vi "FromBaseToMicro.vi"(11 "base":dbl) -> (3 "u":dbl format="%#_13g")   [LabVIEW 2014]
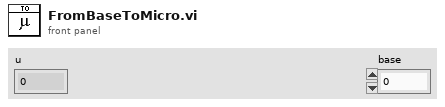
[diagram p1: front panel]
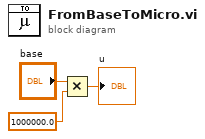
[diagram p0: block diagram]
diagram:
  n1 = Multiply(x="base", y=1000000.0) -> (x*y=→"u":dbl)
